vi "CrossCorr_v1.vi"(1 "Trace2":i32[](array[numeric])=[1, 2, 6, 0, 0, 2, 1, 0, 1, 2, 0, 1, 4, 6, 1], 2 "Trace1":i32[](array[numeric])=[1, 2, 6, 0, 0, 2, 1, 0, 1, 2, 0, 1, 4, 6, 1]) -> (0 "G1-G8":dbl[](array[numeric])=[2139042829303808.0, 2141692421472256.0, 2159988445282304.0, 2136790790045696.0, 2133389444382720.0, 2172897237925888.0, 2132249264783360.0, 2137461610250240.0] format="%.6f")   [LabVIEW 2009]
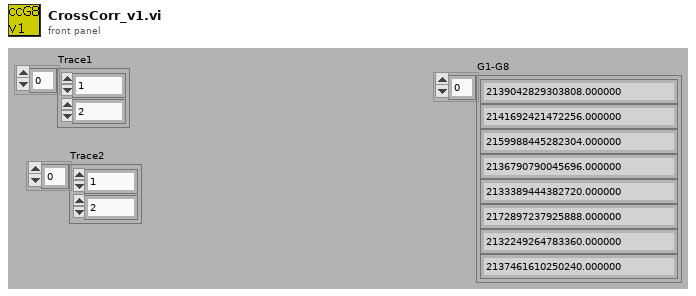
[diagram p1: front panel]
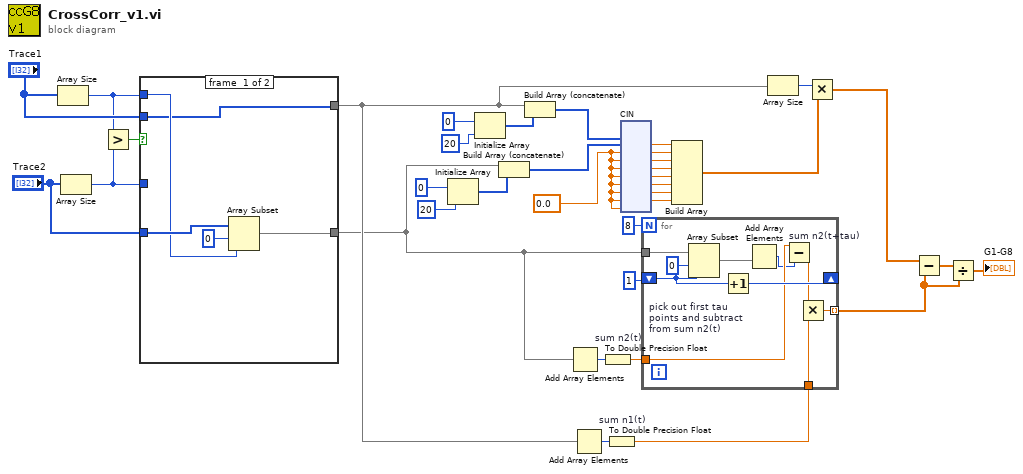
[diagram p0: block diagram]
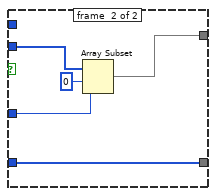
[diagram p2: hidden frame]
diagram:
  w36 = sgl 0.0
  n1 = Array Size(array="Trace1") -> (size(s)=w10:i32)
  n2 = Array Size(array="Trace2") -> (size(s)=w11:i32)
  n3 = Greater?(x=w10, y=w11) -> (0:w14:bool)
  n4 = case shown="True" w14 {
    tunnel: "Trace1" -> [w37 w46]
    tunnel: "Trace2" -> [w40 w42]
    tunnel: w11 -> [_ w44]
    tunnel: [w37 w43] -> w6
    tunnel: [w38 w42] -> w4
    tunnel: w10 -> [w39 _]
    frame #0 {
      n5 = Array Subset(array=w40, index=0, length=w39) -> (w38:i32[])
    }
    frame #1 {
      n6 = Array Subset(array=w46, index=0, length=w44) -> (w43:i32[])
    }
  }
  n7 = Initialize Array(0 ("element"), 20 ("dimension size")) -> (w8:i32[])
  n8 = Initialize Array(0 ("element"), 20 ("dimension size")) -> (w23:i32[])
  n9 = Build Array (concatenate)(w4, w8) -> (w7:i32[])
  n10 = Build Array (concatenate)(w6, w23) -> (w24:i32[])
  n11 = Add Array Elements(numeric array=w4) -> (sum=w5:i32)
  n12 = Add Array Elements(numeric array=w6) -> (sum=w17:i32)
  n13 = To Double Precision Float "sum n2(t)"(number=w5) -> (double precision float=w2:dbl)
  n14 = To Double Precision Float "sum n1(t)"(number=w17) -> (double precision float=w1:dbl)
  n15 = cin(w24, w7, w36, w36, w36, w36, w36, w36, w36, w36) -> (w35:sgl, w34:sgl, w33:sgl, w32:sgl, w31:sgl, w30:sgl, w29:sgl, w28:sgl)  [unwired: 2 in]
  n16 = for {
    N: 8 -> [_]
    tunnel: w4 -> [w55]
    shift-right: [w56] -> _
    shift-left: 1 ("index") -> [w52]
    tunnel: w2 -> [w51]
    tunnel: [w54] -> w16 mode=indexing
    tunnel: w1 -> [w47]
    n17 = Array Subset "pick out first tau\npoints and subtract\nfrom sum n2(t)"(array=w55, index=0, length=w52) -> (w48:i32[])
    n18 = Increment(x=w52) -> (x+1=w56:i32)
    n19 = Add Array Elements(numeric array=w48) -> (sum=w50:i32)
    n20 = Subtract "sum n2(t+tau)"(x=w51, y=w50) -> (x-y=w49:dbl)
    n21 = Multiply(x=w49, y=w47) -> (x*y=w54:dbl)
  }
  n22 = Build Array(w35, w34, w33, w32, w31, w30, w29, w28) -> (w18:sgl[])
  n23 = Array Size(array=w6) -> (size(s)=w19:i32)
  n24 = Multiply(x=w19, y=w18) -> (x*y=w15:sgl[])
  n25 = Subtract(x=w15, y=w16) -> (x-y=w21:dbl[])
  n26 = Divide(x=w21, y=w16) -> (x/y=→"G1-G8":dbl[])
